vi "uTTA_CreateCAL_File.vi"(4 "error in":errorcluster, 5 "Ext. called":bool, 6 "Ext. File Path":path) -> (0 "error out":errorcluster)   [LabVIEW 2021]
uses:
  SubVi/CTL_uTTA_BlockDiagCal.ctl
  uTTA_Device_Driver/uTTA_Controls/CTL_uTTA_TSP_Calibration.ctl
  uTTA_Device_Driver/uTTA_Controls/CTL_uTTA_TSP_CalStatus.ctl
  <vilib>/Utility/miscctls.llb/LVPointTypeDef.ctl
panel:
  in  "Tab Control":T1(tab)
  in  "uTTA Calibration":T2 {"I_Sense Offset" format="%#3.3pA"; "I_Sense Gain" format="%#3.3pA/Digit"; "CH_I Offset" format="%#3.3pA"; "CH_I Gain" format="%#3.3pA/Digit"; "CH0 PA3 Offset" format="%#3.3pV"; "CH0 PA3 Gain" format="%#3.3pV/Digit"; "CH0 PA2 Offset" format="%#3.3pV"; "CH0 PA2 Gain" format="%#3.3pV/Digit"; "CH0 PA1 Offset" format="%#3.3pV"; "CH0 PA1 Gain" format="%#3.3pV/Digit"; "CH0 PA0 Offset" format="%#3.3pV"; "CH0 PA0 Gain" format="%#3.3pV/Digit"; "CH3 PA0 Offset" format="%#3.3pV"; "CH3 PA0 Gain" format="%#3.3pV/Digit"; "CH2 PA0 Offset" format="%#3.3pV"; "CH2 PA0 Gain" format="%#3.3pV/Digit"; "CH1 PA0 Offset" format="%#3.3pV"; "CH1 PA0 Gain" format="%#3.3pV/Digit"; "Voffs1 Offset" format="%#3.3pV"; "Voffs1 Gain" format="%#3.3pV/Digit"; "Voffs0 Offset" format="%#3.3pV"; "CH3 Diff Gain" format="%#3.3pV/V"; "CH2 Diff Gain" format="%#3.3pV/V"; "CH1 Diff Gain" format="%#3.3pV/V"; "Voffs0 Gain" format="%#3.3pV/Digit"; "CH0 Diff Gain" format="%#3.3pV/V"}
  in  "TSP Channels":T3 {"Offset" format="%.3pV"; "Lin. Gain" format="%#.4pV/K"; "Quad. Gain" format="%.5pV/K²"}
  in  "TC Channels":T5(array[cluster]) {"Offset" format="%.2p°C"; "Lin. Gain" format="%#.3p°C/K"; "Quad. Gain" format="%.3p°C/K²"}
  in  "DeviceInfo":string[][](array[string])
  in  "Read uTTA-Cal":bool
  in  "Write uTTA-Cal":bool
  in  "Exit":bool
  # "G0"
  # "G1"
  # "G2"
  # "G3"
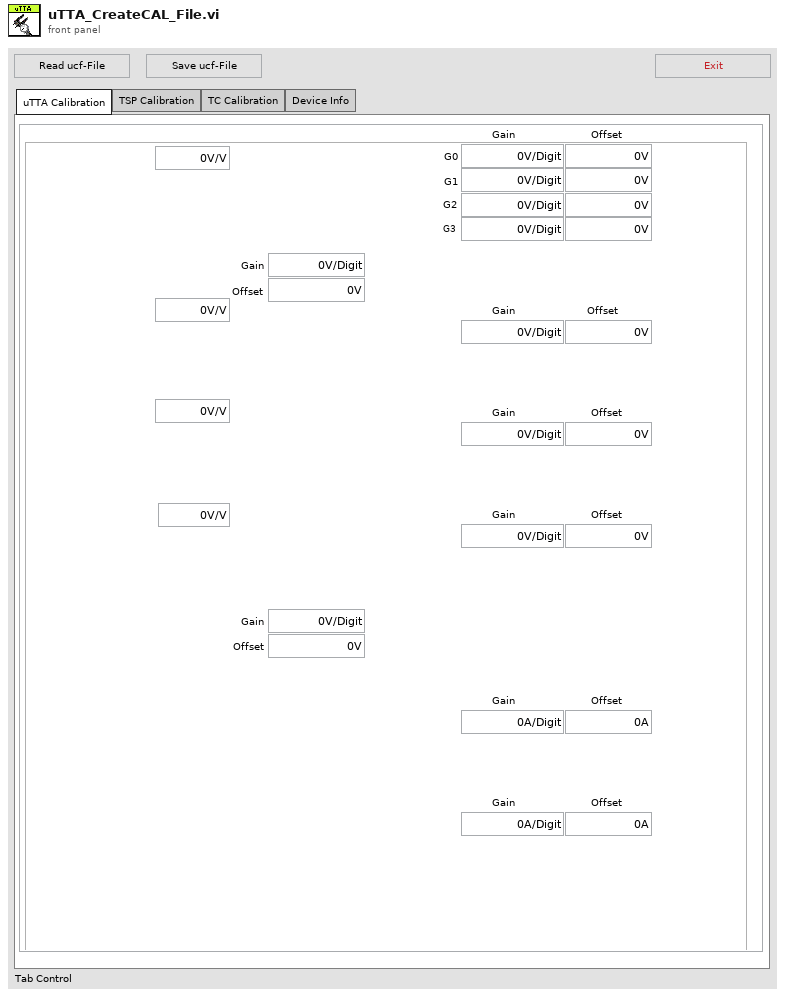
[diagram p1: front panel]
types:
  T1 = enum32{"uTTA Calibration", "TSP Calibration", "TC Calibration", "Device Info"}
  T2 = typedef "CTL_uTTA_BlockDiagCal.ctl" = cluster{"CH0 Diff Gain":dbl, "Voffs0 Gain":dbl, "CH1 Diff Gain":dbl, "CH2 Diff Gain":dbl, "CH3 Diff Gain":dbl, "Voffs0 Offset":dbl, "Voffs1 Gain":dbl, "Voffs1 Offset":dbl, "CH1 PA0 Gain":dbl, "CH1 PA0 Offset":dbl, "CH2 PA0 Gain":dbl, "CH2 PA0 Offset":dbl, "CH3 PA0 Gain":dbl, "CH3 PA0 Offset":dbl, "CH0 PA0 Gain":dbl, "CH0 PA0 Offset":dbl, "CH0 PA1 Gain":dbl, "CH0 PA1 Offset":dbl, "CH0 PA2 Gain":dbl, "CH0 PA2 Offset":dbl, "CH0 PA3 Gain":dbl, "CH0 PA3 Offset":dbl, "CH_I Gain":dbl, "CH_I Offset":dbl, "I_Sense Gain":dbl, "I_Sense Offset":dbl}
  T3 = typedef "CTL_uTTA_TSP_Calibration.ctl" = cluster{"Channel Name":string, "Offset":dbl, "Lin. Gain":dbl, "Quad. Gain":dbl, "Cal Status":T4}[]
  T4 = typedef "CTL_uTTA_TSP_CalStatus.ctl" = enum16{"Uncalibrated", "Calibrated", "Dummy"}
  T5 = cluster{"Channel Name":string, "Offset":dbl, "Lin. Gain":dbl, "Quad. Gain":dbl}[]
  T6 = typedef "LVPointTypeDef.ctl" = cluster{"Horizontal":i16, "Vertical":i16}
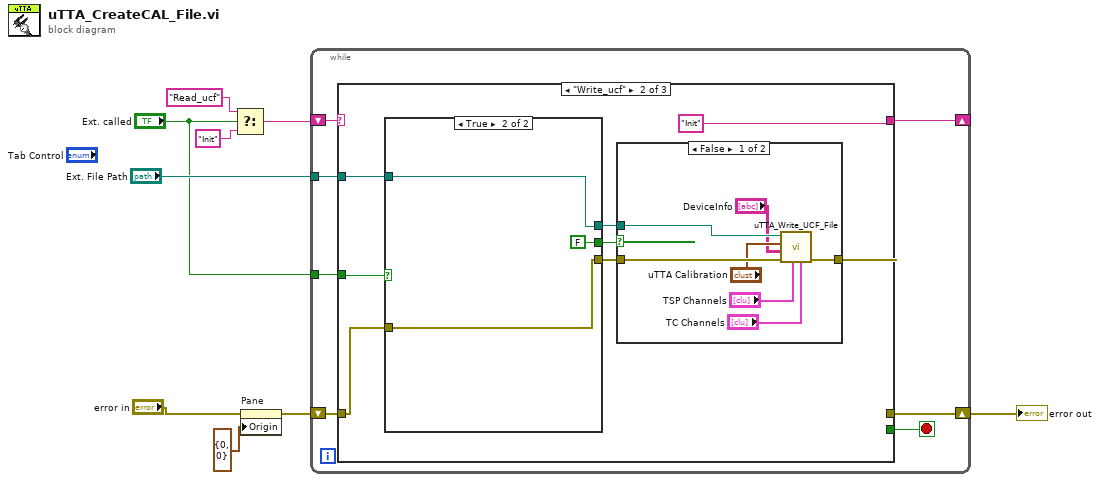
[diagram p0: block diagram]
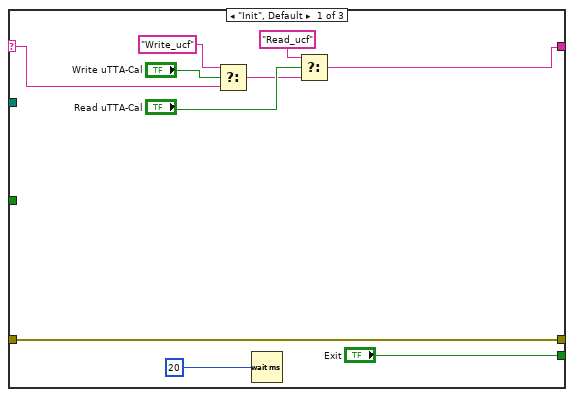
[diagram p2: hidden frame]
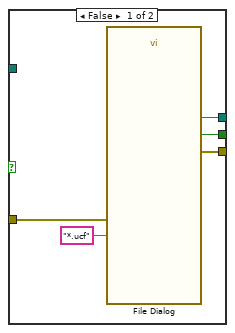
[diagram p3: hidden frame]
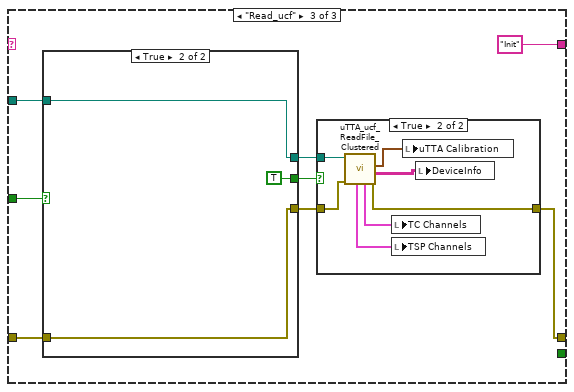
[diagram p5: hidden frame]
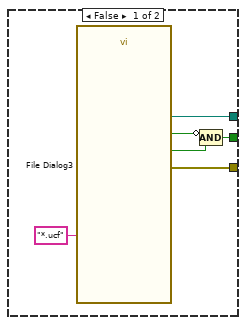
[diagram p6: hidden frame]
diagram:
  n1 = Select(t="Read_ucf", s="Ext. called", f="Init" ("pattern (all files)")) -> (s? t:f=w4:string)
  n2 = property on="Pane" class="Pane"(error in="error in", "Origin"=T6 {"Horizontal"=0, "Vertical"=0}) -> (error out=w9:errorcluster)  [unwired: 1 in, 1 out]
  n3 = while {
    shift-right: [w15] -> _
    shift-left: w4 -> [w16]
    shift-right: [w12] -> w6
    shift-left: w9 -> [w13]
    tunnel: "Ext. File Path" -> [w11]
    tunnel: "Ext. called" -> [w10]
    stop <- w14 stop-if-true
    n4 = case shown="\"Write_ucf\"" w16 {
      selector: w16 -> [w24 _ _]
      tunnel: [w20 "Init" ("pattern (all files)") "Init" ("pattern (all files)")] -> w15
      tunnel: ["Exit" _ _] -> w14
      tunnel: w13 -> [w17 w30 w53]
      tunnel: [w17 w29 w52] -> w12
      tunnel: w11 -> [_ w27 w51]
      tunnel: w10 -> [_ w28 w54]
      frame "Init", Default {
        n5 = Select(t="Write_ucf", s="Write uTTA-Cal", f=w24) -> (s? t:f=w18:string)
        n6 = Wait (ms)(milliseconds to wait=u32 20) -> ()  [unwired: 1 out]
        n7 = Select(t="Read_ucf", s="Read uTTA-Cal", f=w18) -> (s? t:f=w20:string)
      }
      frame "Write_ucf" {
        n8 = case shown="True" w28 {
          tunnel: [w39 FALSE ("cancelled")] -> w34
          tunnel: [w38 w42] -> w33
          tunnel: [w37 w40] -> w32
          tunnel: w30 -> [w35 w42]
          tunnel: w27 -> [_ w40]
          frame False {
            n9 = call "File Dialog"("error in"=w35, "pattern (all files)"="*.ucf") -> ("selected path"=w37:path, "cancelled"=w39:bool, "error out"=w38:errorcluster)  [unwired: 10 in, 1 out]
          }
          frame True {
          }
        }
        n10 = case shown="False" w34 {
          tunnel: w33 -> [w48 w50]
          tunnel: w32 -> [w49 _]
          tunnel: [w47 w50] -> w29
          frame False {
            n11 = call "uTTA_Write_UCF_File.vi"("TC_Channels"="TC Channels", "TSP_Channels"="TSP Channels", "error in (no error)"=w48, "DeviceInfo"="DeviceInfo", "Inputs"="uTTA Calibration", "selected path"=w49) -> ("error out"=w47:errorcluster)  [unwired: 4 in, 1 out]
          }
          frame True {
          }
        }
      }
      frame "Read_ucf" {
        n12 = case shown="True" w54 {
          tunnel: [w64 w66] -> w58
          tunnel: [w63 w65] -> w57
          tunnel: [w59 TRUE] -> w55
          tunnel: w53 -> [_ w66]
          tunnel: w51 -> [_ w65]
          frame False {
            n13 = call "File Dialog3"("pattern (all files)"="*.ucf") -> ("selected path"=w63:path, "exists"=w61:bool, "cancelled"=w60:bool, "error out"=w64:errorcluster)  [unwired: 11 in]
            n14 = Compound Arithmetic op=AND(invert w60, w61) -> (w59:bool)
          }
          frame True {
          }
        }
        n15 = case shown="True" w55 {
          tunnel: w58 -> [w68 w74]
          tunnel: w57 -> [_ w75]
          tunnel: [w68 w73] -> w52
          frame False {
          }
          frame True {
            n16 = call "uTTA_ucf_ReadFile_Clustered.vi"("error in (no error)"=w74, "selected path"=w75) -> ("error out"=w73:errorcluster, "DeviceInfo"=w69:string[][], "uTTA_Cal"=w72:T2, "TC_Channels"=w71:T5, "TSP_Channels"=w70:T3)  [unwired: 4 in, 1 out]
            n17 = local write "TC Channels"(w71) -> ()
            n18 = local write "TSP Channels"(w70) -> ()
            n19 = local write "uTTA Calibration"(w72) -> ()
            n20 = local write "DeviceInfo"(w69) -> ()
          }
        }
      }
    }
  }
  "error out" <- w6
